vi "DAQmx Read (Power Wfm 1Chan NSamp).vi"(0 "task/channels in":refnum<k21>, 7 "number of samples per channel":i32=-1, 9 "timeout":dbl=10.0 format="%0.2f", 11 "error in":errorcluster) -> (4 "task out":refnum<k21>, 6 "voltage":waveform(dbl), 8 "current":waveform(dbl), 15 "error out":errorcluster)   [LabVIEW 2024]
doc: "Reads a waveform that contains one or more floating-point samples from a task that contains a single power channel."
uses:
  nilvaiu.dll
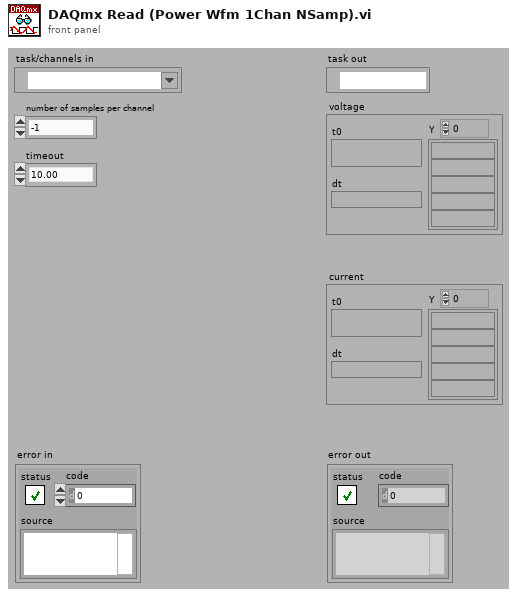
[diagram p1: front panel]
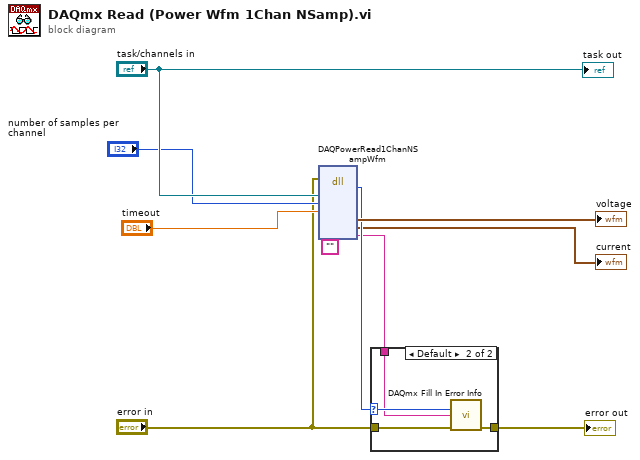
[diagram p0: block diagram]
diagram:
  n1 = dll-call lib="nilvaiu.*" fn="DAQPowerRead1ChanNSampWfm"(error in="error in", "taskID"="task/channels in", "numberOfSamples"="number of samples per channel", "timeout"="timeout", "extendedErrorInfo"="") -> ("return type"=w5:i32, "voltage"=→"voltage":waveform(dbl), "current"=→"current":waveform(dbl), "extendedErrorInfo"=w3:string)  [unwired: 4 in, 5 out]
  n2 = case shown="Default" w5 {
    selector: w5 -> [_ w13]
    tunnel: "error in" -> [w11 w15]
    tunnel: [w11 w14] -> w10
    tunnel: w3 -> [_ w12]
    frame 0 {
    }
    frame Default {
      n3 = call "DAQmx Fill In Error Info.vi"("status code"=w13, "extended error info"=w12, "error in"=w15) -> ("error out"=w14:errorcluster)  [unwired: 1 in, 11 out]
    }
  }
  "error out" <- w10
  "task out" <- "task/channels in"
